vi "debugg app.vi"() -> ()   [LabVIEW 2013]
panel:
  in  "stop":bool
  out "Thermometer K":dbl(slide) scale=280.0..330.0
  out "Thermometer stC":dbl(slide) scale=0.0..100.0
  out "Waveform Chart":dbl(graph)
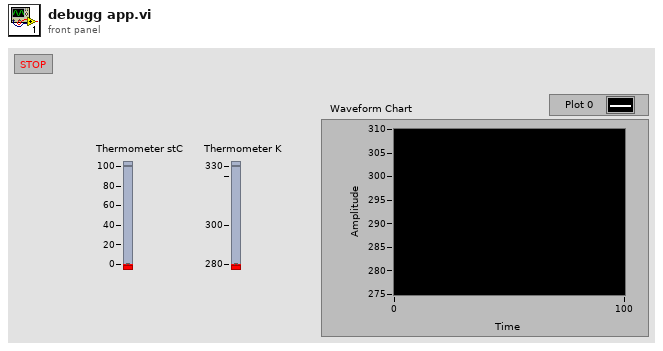
[diagram p1: front panel]
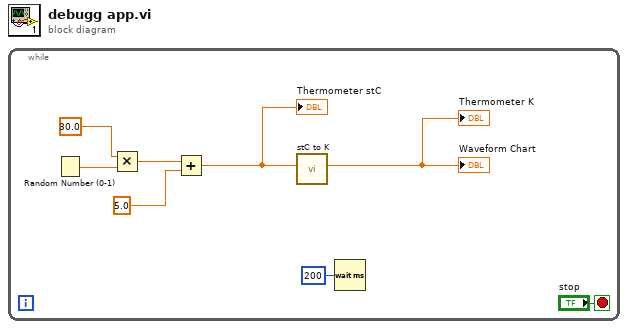
[diagram p0: block diagram]
diagram:
  n1 = while {
    stop <- "stop" stop-if-true
    n2 = Random Number (0-1)() -> (number: 0 to 1=w5:dbl)
    n3 = Multiply(x=30.0 ("a"), y=w5) -> (x*y=w8:dbl)
    n4 = Add(x=w8, y=5.0 ("b")) -> (x+y=w1:dbl)
    "Thermometer stC" <- w1
    n5 = call "stC to K.vi"("stC (0)"=w1) -> ("K"=→"Waveform Chart" →"Thermometer K":dbl)  [unwired: 9 in, 1 out]
    n6 = Wait (ms)(milliseconds to wait=u32 200) -> ()  [unwired: 1 out]
  }
